vi "Locate-Done.vi"(7 "InputString":string, 13 "Char":string) -> (8 "Boolean":bool)   [LabVIEW 2011]
panel:
  out "match substring":string
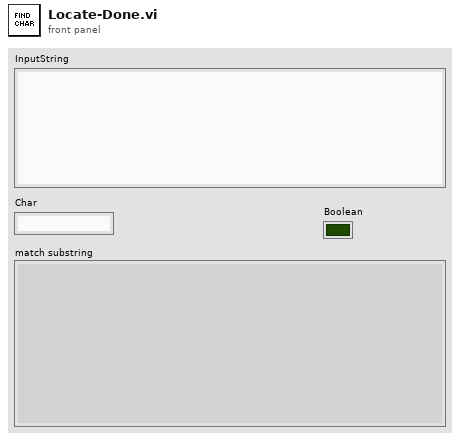
[diagram p1: front panel]
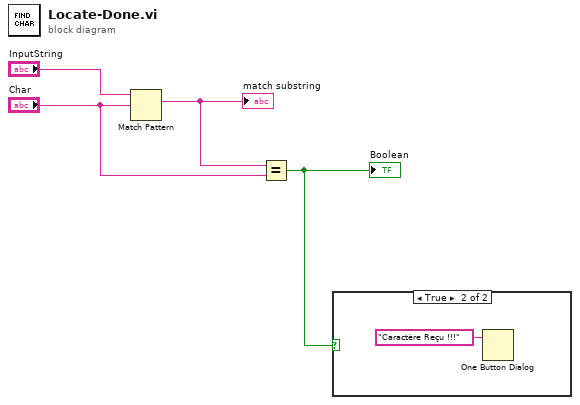
[diagram p0: block diagram]
diagram:
  n1 = Match Pattern(string="InputString", regular expression="Char") -> (match substring=w4:string)  [unwired: 1 in, 3 out]
  "match substring" <- w4
  n2 = Equal?(x=w4, y="Char") -> (x = y?=w1:bool)
  "Boolean" <- w1
  n3 = case shown="True" w1 {
    frame False {
    }
    frame True {
      n4 = One Button Dialog(message="Caractère Reçu !!!") -> ()  [unwired: 1 in, 1 out]
    }
  }
